vi "A170316-11_IO.vi"() -> ()   [LabVIEW 2020]
panel:
  in  "选项卡控件":enum32{"数字量输入", "数字量输出", "模拟量/伺服"}(tab)
  out "I 0":T1
  out "I 1":T2
  out "I 2":T3
  out "I 3":T4
  in  "Q 0":T5
  in  "Q 1":T6
  # "总成检验"
  # "/"
  # "蜗杆伺服"
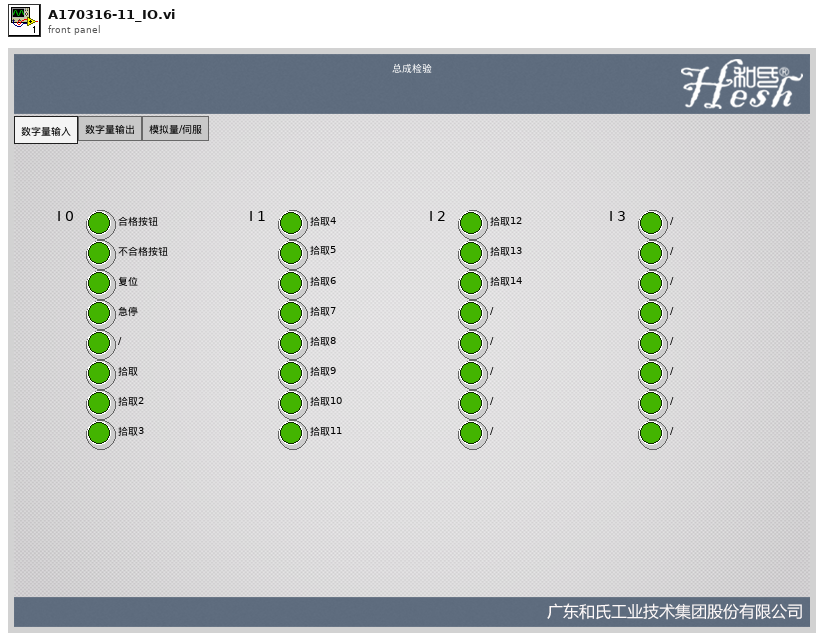
[diagram p1: front panel]
types:
  T1 = cluster{"合格按钮":bool, "不合格按钮":bool, "复位":bool, "急停":bool, "/":bool, "拾取":bool, "拾取2":bool, "拾取3":bool}
  T2 = cluster{"拾取4":bool, "拾取5":bool, "拾取6":bool, "拾取7":bool, "拾取8":bool, "拾取9":bool, "拾取10":bool, "拾取11":bool}
  T3 = cluster{"拾取12":bool, "拾取13":bool, "拾取14":bool, "/":bool, "/":bool, "/":bool, "/":bool, "/":bool}
  T4 = cluster{"/":bool, "/":bool, "/":bool, "/":bool, "/":bool, "/":bool, "/":bool, "/":bool}
  T5 = cluster{"蜗杆伺服脉冲A":bool, "蜗杆伺服脉冲B":bool, "三色灯-红":bool, "三色灯-黄":bool, "三色灯-绿":bool, "三色灯-蜂鸣器":bool, "合格指示灯":bool, "不合格指示灯":bool}
  T6 = cluster{"/":bool, "备用1":bool, "备用2":bool, "备用3":bool, "/":bool, "/":bool, "/":bool, "/":bool}
  T7 = cluster{"[0]":bool, "[1]":bool, "[2]":bool, "[3]":bool, "[4]":bool, "[5]":bool, "[6]":bool, "[7]":bool}
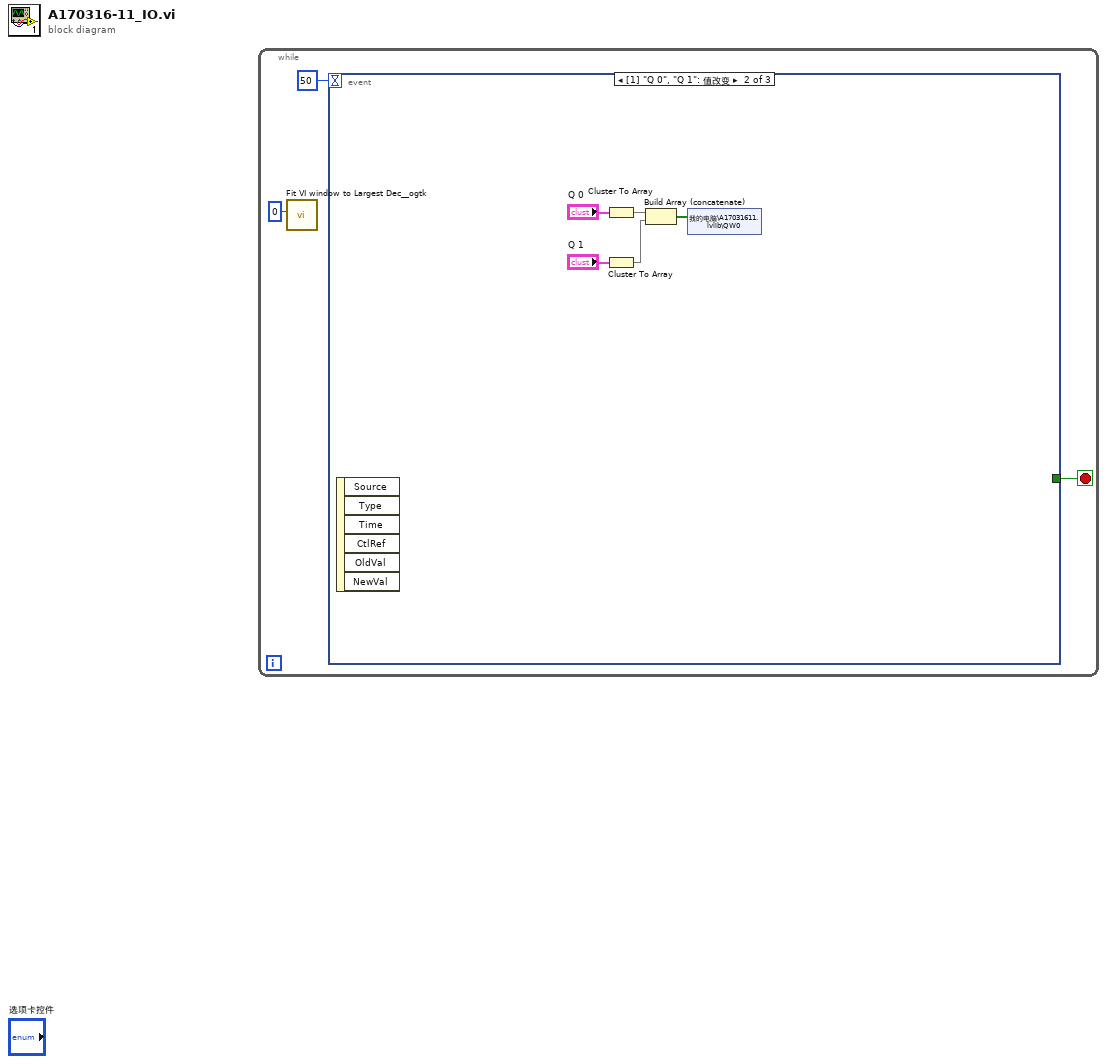
[diagram p0: block diagram]
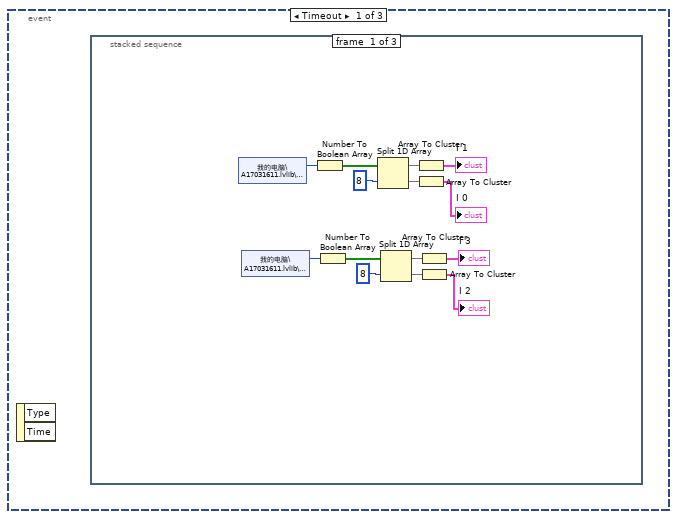
[diagram p2: hidden frame]
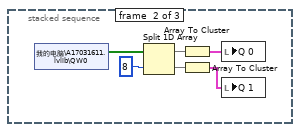
[diagram p3: hidden frame]
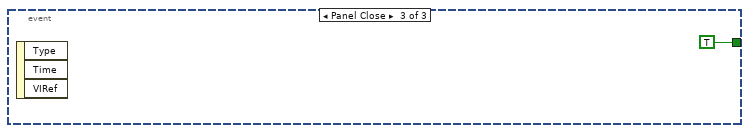
[diagram p5: hidden frame]
diagram:
  n1 = while {
    stop <- w3 stop-if-true
    n2 = call <userlib>:"Fit VI window to Largest Dec__ogtk.vi"("border spacing (2 px)"=0) -> ()  [unwired: 5 in, 2 out]
    n3 = event shown="[1] \"Q 0\", \"Q 1\": 值改变" {
      selector: _ -> [_ _ _]
      dyn-events: _ -> [_ _ _]
      timeout: 50 -> [_ _ _]
      tunnel: [_ _ TRUE] -> w3
      event Timeout {
        n4 = event-data() -> ()  [unwired: 1 in, 2 out]
        n5 = stacked-sequence {
          frame #0 {
            n6 = shared-variable "我的电脑\\A17031611.lvlib\\IW0"() -> (w15:u16)  [unwired: 1 in, 1 out]
            n7 = shared-variable "我的电脑\\A17031611.lvlib\\IW2"() -> (w14:u16)  [unwired: 1 in, 1 out]
            n8 = Number To Boolean Array(number=w15) -> (Boolean array=w17:bool[])
            n9 = Number To Boolean Array(number=w14) -> (Boolean array=w16:bool[])
            n10 = Split 1D Array(array=w17, index=8 ("索引")) -> (first subarray=w13:bool[], second subarray=w10:bool[])
            n11 = Split 1D Array(array=w16, index=8 ("索引")) -> (first subarray=w11:bool[], second subarray=w12:bool[])
            n12 = Array To Cluster(array=w13) -> (cluster=→"I 1":T7)
            n13 = Array To Cluster(array=w10) -> (cluster=→"I 0":T7)
            n14 = Array To Cluster(array=w11) -> (cluster=→"I 3":T7)
            n15 = Array To Cluster(array=w12) -> (cluster=→"I 2":T7)
          }
          frame #1 {
            n16 = shared-variable "我的电脑\\A17031611.lvlib\\QW0"() -> (w23:bool[])  [unwired: 1 in, 1 out]
            n17 = Split 1D Array(array=w23, index=8 ("索引")) -> (first subarray=w21:bool[], second subarray=w20:bool[])
            n18 = Array To Cluster(array=w21) -> (cluster=w19:T7)
            n19 = Array To Cluster(array=w20) -> (cluster=w18:T7)
            n20 = local write "Q 0"(w19) -> ()
            n21 = local write "Q 1"(w18) -> ()
          }
          frame #2 {
          }
        }
      }
      event "Q 0", "Q 1": Value Change {
        n22 = event-data() -> ()  [unwired: 1 in, 6 out]
        n23 = Cluster To Array(cluster="Q 0") -> (array=w26:bool[])
        n24 = Cluster To Array(cluster="Q 1") -> (array=w25:bool[])
        n25 = Build Array (concatenate)(w26, w25) -> (w24:bool[])
        n26 = shared-variable "我的电脑\\A17031611.lvlib\\QW0"(w24) -> ()  [unwired: 1 in, 1 out]
      }
      event Panel Close {
        n27 = event-data() -> ()  [unwired: 1 in, 3 out]
      }
    }
  }
